vi "Gas Heater Test.vi"(8 "error in":errorcluster) -> (0 "error out":errorcluster)   [LabVIEW 2015]
uses:
  CAN Communication/Peltier/Typedefs/Peltier Temperature Sensors.ctl
  CAN Communication/Peltier/Peltier.lvclass
  CAN Communication/Gas/Gas.lvclass
panel:
  out "Pass":bool
  in  "Stop":bool
  out "TS5":dbl
  out "Timeout":i32
  out "Error":errorcluster
  # "Gas Heater Test"
  # "This test performs functionality\ntesting on the Gas Heater.\n\nPlease standby while the test is\nin progress..."
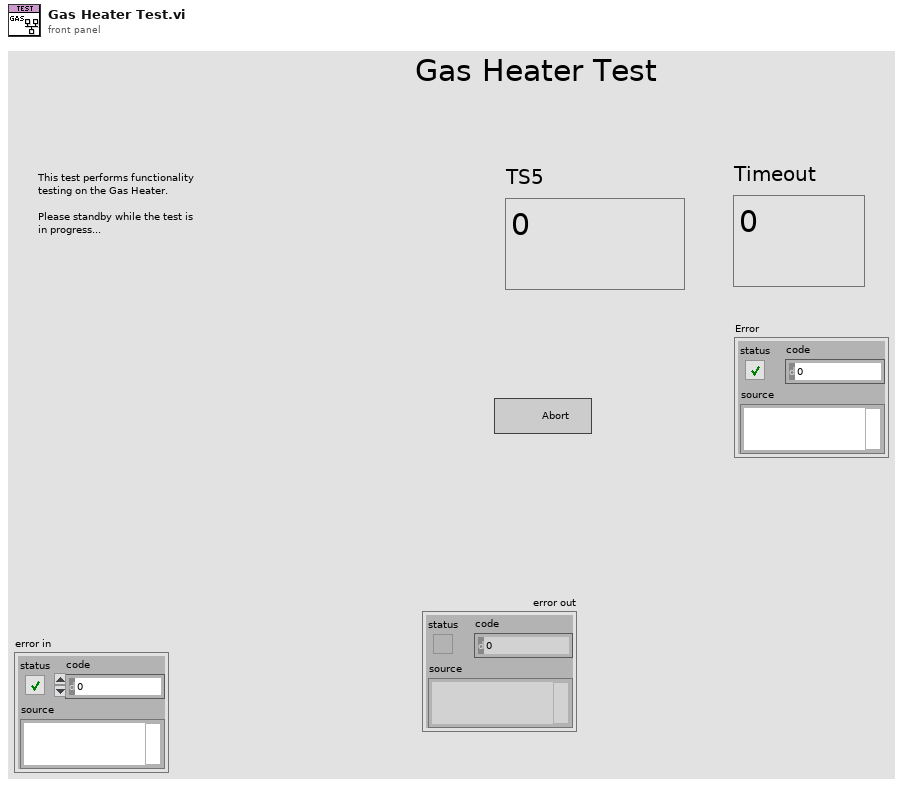
[diagram p1: front panel]
types:
  T1 = typedef "Peltier.lvclass/Peltier Temperature Sensors.ctl" = u16
  T2 = typedef "Gas.lvclass/Session Handle.ctl" = refnum<data-value>
  T3 = typedef "User Configuration.ctl" = cluster{"Password":string, "cDAQ Name":string, "CAN Interface":string}
  T4 = typedef "Peltier.lvclass/Session Handle.ctl" = refnum<data-value>
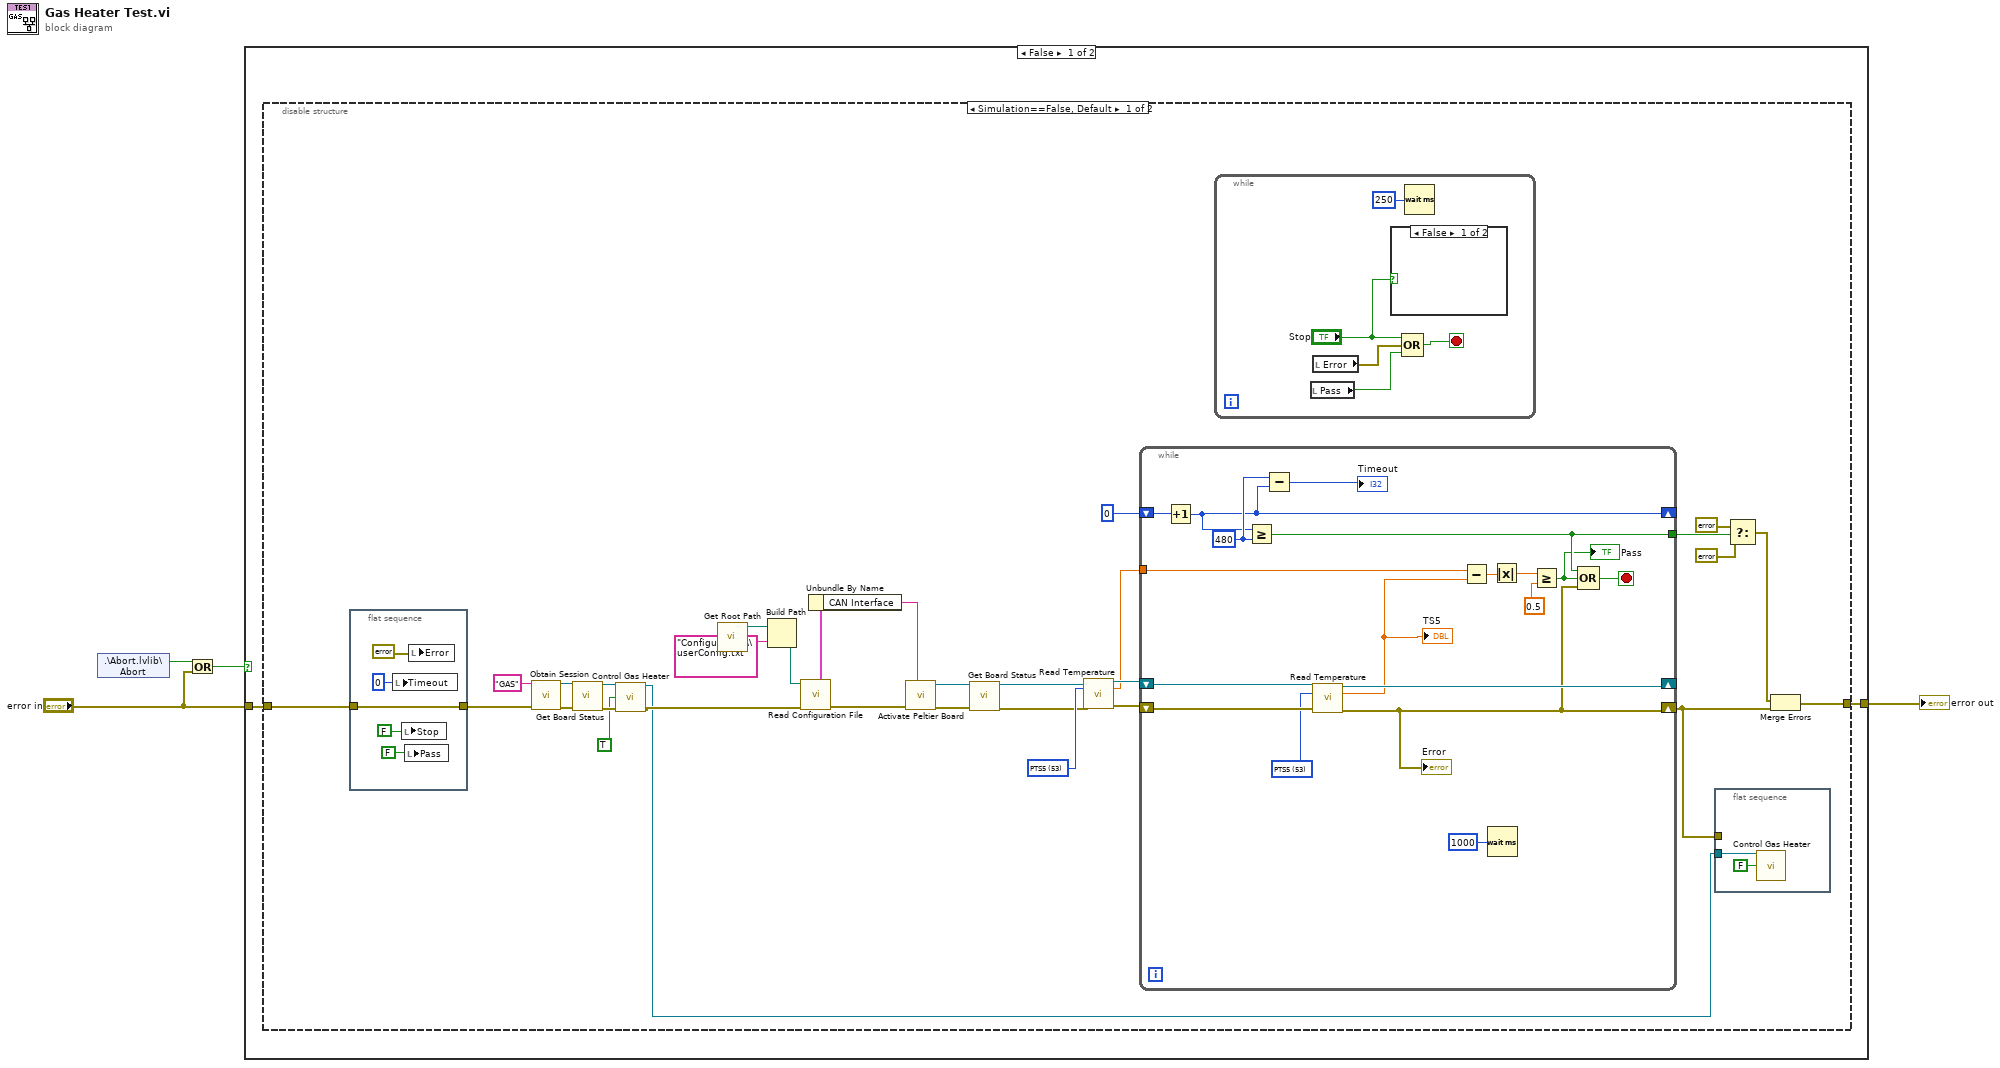
[diagram p0: block diagram]
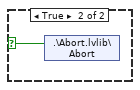
[diagram p2: hidden frame]
diagram:
  n1 = shared-variable ".\\Abort.lvlib\\Abort"() -> (w3:bool)  [unwired: 1 in, 1 out]
  n2 = Or(x=w3, y="error in") -> (x .or. y?=w1:bool)
  n3 = case shown="False" w1 {
    tunnel: [w6 w70] -> w4
    tunnel: "error in" -> [w5 w70]
    frame False {
      n4 = disable-structure shown="Simulation==False, Default" {
        disable-tunnel: [w28 w69] -> w6
        disable-tunnel: w5 -> [w22 w69]
        frame condition #0 (active) {
          w35 = T1 53 items=["PTS1"=49, "PTS2"=50, "PTS3"=51, "PTS4"=52, "PTS5"=53, "PTS6"=54] ("Pelt Temp Sensors")
          n5 = flat-sequence {
            tunnel: [w44] -> w21
            tunnel: w22 -> [w44]
            frame #0 {
              n6 = local write "Timeout"(0 ("Timeout")) -> ()
              n7 = local write "Stop"(FALSE ("Stop")) -> ()
              n8 = local write "Pass"(FALSE ("Pass")) -> ()
              n9 = local write "Error"(errorcluster {"status"=FALSE, "code"=0, "source"=""} ("Peltier Errors")) -> ()
            }
          }
          n10 = call "Obtain Session.vi"("Session  Name ()"="GAS", "error in (no error)"=w21) -> ("Session Handle"=w19:T2, "error out"=w20:errorcluster)  [unwired: 12 in]
          n11 = call "Get Board Status.vi"("Session Handle in"=w19, "error in (no error)"=w20) -> ("Session Handle out"=w26:T2, "error out"=w25:errorcluster)  [unwired: 11 in, 1 out]
          n12 = call "Control Gas Heater.vi"("Session Handle in"=w26, "On?"=TRUE, "error in (no error)"=w25) -> ("Session Handle out"=w8:T2, "error out"=w12:errorcluster)  [unwired: 10 in, 1 out]
          n13 = call "Get Root Path.vi"() -> ("Root Path"=w15:path)  [unwired: 11 in]
          n14 = Build Path(base path=w15, name or relative path="Configuration\\userConfig.txt") -> (appended path=w17:path)
          n15 = call "Read Configuration File.vi"("error in (no error)"=w12, "Filepath"=w17) -> ("error out"=w16:errorcluster, "User Config"=w14:T3)  [unwired: 8 in]
          n16 = Unbundle By Name(w14) -> ("CAN Interface"=w13:string)
          n17 = call "Activate Peltier Board.vi"("CAN Interface"=w13, "error in (no error)"=w16) -> ("error out"=w10:errorcluster, "Session Handle Out"=w11:T4)  [unwired: 8 in]
          n18 = call "Get Board Status.vi"("Session Handle"=w11, "error in (no error)"=w10) -> ("Session Handle Out"=w23:T4, "error out"=w7:errorcluster)  [unwired: 11 in, 1 out]
          n19 = call "Read Temperature.vi"("Session Handle"=w23, "Pelt Temp Sensors"=w35, "error in (no error)"=w7) -> ("Session Handle Out"=w36:T4, "Temperature"=w34:dbl, "error out"=w37:errorcluster)  [unwired: 10 in]
          n20 = while {
            shift-right: [w67] -> _
            shift-left: w36 -> [w55]
            shift-right: [w62] -> w9
            shift-left: w37 -> [w54]
            tunnel: w34 -> [w66]
            shift-right: [w57] -> _
            shift-left: 0 -> [w60]
            tunnel: [w59] -> w29
            stop <- w61 stop-if-true
            w53 = T1 53 items=["PTS1"=49, "PTS2"=50, "PTS3"=51, "PTS4"=52, "PTS5"=53, "PTS6"=54] ("Pelt Temp Sensors")
            w58 = 480 ("y")
            n21 = Increment(x=w60) -> (x+1=w57:i32)
            n22 = Greater Or Equal?(x=w57, y=w58) -> (x >= y?=w59:bool)
            n23 = Subtract(x=w58, y=w57) -> (x-y=→"Timeout":i32)
            n24 = call "Read Temperature.vi"("Session Handle"=w55, "Pelt Temp Sensors"=w53, "error in (no error)"=w54) -> ("Session Handle Out"=w67:T4, "Temperature"=w52:dbl, "error out"=w62:errorcluster)  [unwired: 10 in]
            "Error" <- w62
            "TS5" <- w52
            n25 = Subtract(x=w66, y=w52) -> (x-y=w65:dbl)
            n26 = Wait (ms)(milliseconds to wait=u32 1000) -> ()  [unwired: 1 out]
            n27 = Absolute Value(x=w65) -> (abs(x)=w64:dbl)
            n28 = Greater Or Equal?(x=w64, y=0.5) -> (x >= y?=w51:bool)
            "Pass" <- w51
            n29 = Compound Arithmetic op=OR(w59, w51, w62) -> (w61:bool)
          }
          n30 = while {
            stop <- w45 stop-if-true
            n31 = local read "Pass"() -> (w46:bool)
            n32 = local read "Error"() -> (w47:errorcluster)
            n33 = case shown="False" "Stop" {
              selector: "Stop" -> [_ w50]
              frame False {
              }
              frame True {
                n34 = shared-variable ".\\Abort.lvlib\\Abort"(w50) -> ()  [unwired: 1 in, 1 out]
              }
            }
            n35 = Compound Arithmetic op=OR("Stop", w47, w46) -> (w45:bool)
            n36 = Wait (ms)(milliseconds to wait=u32 250) -> ()  [unwired: 1 out]
          }
          n37 = flat-sequence {
            tunnel: w9 -> [_]
            tunnel: w8 -> [w39]
            frame #0 {
              n38 = call "Control Gas Heater.vi"("Session Handle in"=w39, "On?"=FALSE) -> ()  [unwired: 11 in, 3 out]
            }
          }
          n39 = Select(t=errorcluster {"status"=TRUE, "code"=9002, "source"="Timeout Error. Gas Heater failed to impact Peltier Temperature Sensor."} ("error out"), s=w29, f=errorcluster {"status"=FALSE, "code"=0, "source"=""} ("error out")) -> (s? t:f=w30:errorcluster)
          n40 = Merge Errors(w30, w9) -> (w28:errorcluster)
        }
        frame condition #1 {
        }
      }
    }
    frame True {
    }
  }
  "error out" <- w4
